vi "Move -- subVI.vi"(8 "error in (no error)":errorcluster, 10 "Wavelength":dbl, 11 "VISA Refnum in":refnum<visa-resource-name>) -> (0 "error out":errorcluster)   [LabVIEW 2020, in "Monochromator.lvlib"]
uses:
  Monochromator.lvlib
  <vilib>/Instr/_visa.llb/VISA Flush IO Buffer Mask.ctl
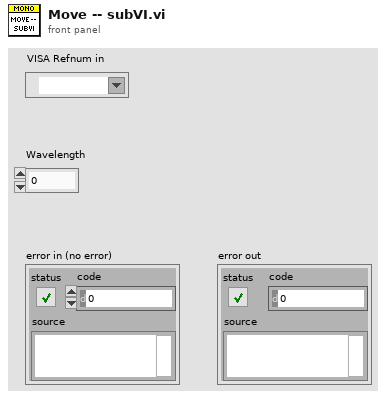
[diagram p1: front panel]
types:
  T1 = typedef "VISA Flush IO Buffer Mask.ctl" = u16
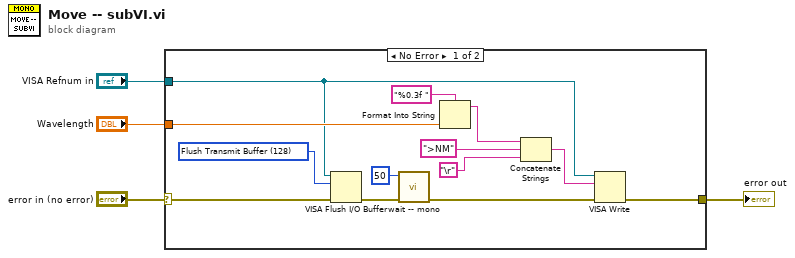
[diagram p0: block diagram]
diagram:
  n1 = case shown="No Error" "error in (no error)" {
    selector: "error in (no error)" -> [w8 w18]
    tunnel: [w17 w18] -> w4
    tunnel: "Wavelength" -> [w14 _]
    tunnel: "VISA Refnum in" -> [w6 _]
    frame No Error {
      w5 = T1 128 items=["Flush Receive Buffer"=16, "Write Transmit Buffer to Device"=32, "Flush Receive Buffer (No I/O)"=64, "Flush Transmit Buffer"=128] ("Mask")
      n2 = VISA Flush I/O Buffer(VISA resource name=w6, mask (16)=w5, error in (no error)=w8) -> (error out=w7:errorcluster)  [unwired: 1 out]
      n3 = call "wait -- mono.vi"("error in (no error)"=w7, "milliseconds to wait"=u32 50) -> ("error out"=w10:errorcluster)  [unwired: 9 in]
      n4 = Format Into String(format string="%0.3f ", w14) -> (resulting string=w16:string)  [unwired: 2 in, 1 out]
      n5 = Concatenate Strings(w16, ">NM" ("string"), "\r") -> (w11:string)
      n6 = VISA Write(VISA resource name=w6, write buffer=w11, error in (no error)=w10) -> (error out=w17:errorcluster)  [unwired: 2 out]
    }
    frame Error {
    }
  }
  "error out" <- w4
